vi "Handle LogRec.vi"(8 "error in":errorcluster, 10 "LogRecord":refnum<class "LogRecord.lvclass">, 11 "UserEventHandler in":refnum<class "UserEventHandler.lvclass">) -> (0 "error out":errorcluster, 3 "UserEventHandler out":refnum<class "UserEventHandler.lvclass">)   [LabVIEW 2020, in "hse-logger.lvlib" / "UserEventHandler.lvclass"]
doc: "Handles the incoming ``LogRecord`` object. If the level of the record is greater or equal to the level of the handler, then a user event is generated with the ``LogRecord`` as payload. \n\n____\nHAMPEL SOFTWARE ENGINEERING v2.0.6 (2021-04-15 11:38)"
uses:
  UserEventHandler.lvclass
  LogRecord/LogRecord.lvclass
  LogRecord/LogRecord.lvclass/LogRecord.ctl
  UserEventHandler.lvclass/UserEventHandler.ctl
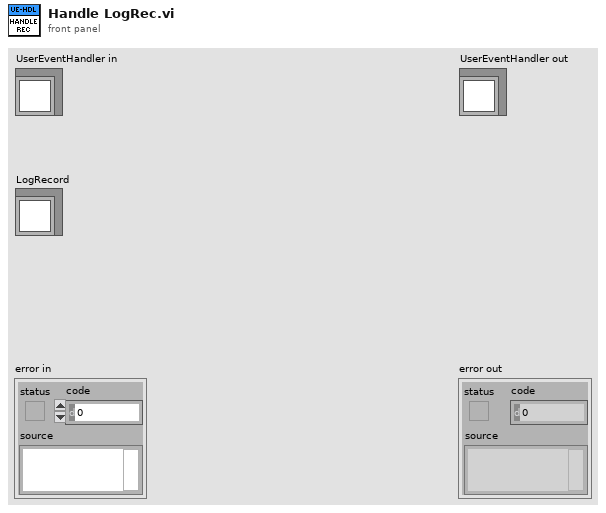
[diagram p1: front panel]
types:
  T1 = typedef "hse-logger.lvlib/LogLevel.ctl" = enum16{"DEBUG", "INFO", "WARNING", "ERROR", "CRITICAL"}
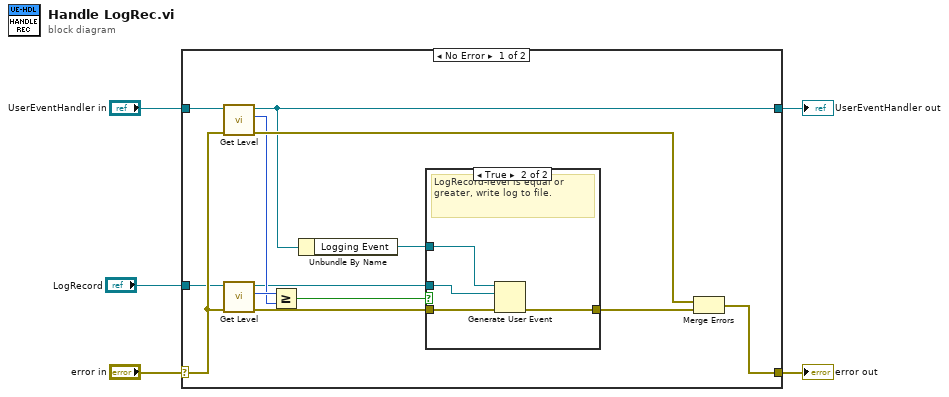
[diagram p0: block diagram]
diagram:
  n1 = case shown="No Error" "error in" {
    selector: "error in" -> [w17 w25]
    tunnel: [w7 w25] -> w4
    tunnel: [w10 w24] -> w2
    tunnel: "UserEventHandler in" -> [w16 w24]
    tunnel: "LogRecord" -> [w15 _]
    frame No Error {
      n2 = call-dynamic "Get Level.vi"("error in"=w17, "Handler in"=w16) -> ("error out"=w18:errorcluster, "Level"=w13:T1, "Handler out"=w10:refnum<class "UserEventHandler.lvclass">)  [unwired: 7 in]
      n3 = call "Get Level.vi"("error in"=w17, "LogRecord in"=w15) -> ("error out"=w11:errorcluster, "Level"=w14:T1, "LogRecord out"=w8:refnum<class "LogRecord.lvclass">)  [unwired: 7 in]
      n4 = Greater Or Equal?(x=w14, y=w13) -> (x >= y?=w12:bool)
      n5 = Unbundle By Name(w10) -> ("Logging Event"=w9:refnum<user-event>)
      n6 = case shown="True" w12 {
        tunnel: w11 -> [w19 w23]
        tunnel: w9 -> [_ w22]
        tunnel: w8 -> [_ w21]
        tunnel: [w19 w20] -> w6
        frame False {
          # "Do not write to file."
        }
        frame True {
          # "LogRecord-level is equal or greater, write log to file."
          n7 = Generate User Event(user event=w22, event data cluster=w21, error in=w23) -> (error out=w20:errorcluster)  [unwired: 1 in, 1 out]
        }
      }
      n8 = Merge Errors(w18, w6) -> (w7:errorcluster)
    }
    frame Error {
    }
  }
  "error out" <- w4
  "UserEventHandler out" <- w2
